vi "Photocell Read.vi"(0 "Arduino Resource":T1={"VISA resource"="", "Board Type"=enum."Arduino Uno", "Connection Type"=enum."USB / Serial", "Bytes Per Packet (15)"=15}, 5 "Photo Cell Pin (0)":u8, 9 "Vcc (5)":dbl=5.0, 11 "error in":errorcluster) -> (4 "Arduino Resource":T1={"VISA resource"="", "Board Type"=enum."Arduino Uno", "Connection Type"=enum."USB / Serial", "Bytes Per Packet (15)"=15}, 8 "Light Intensity (0 - 100)":dbl(knob) scale=0.0..100.0, 15 "error out":errorcluster)   [LabVIEW 2011, in "LabVIEW Interface for Arduino.lvlib"]
doc: "Measure light intensity using a Photocell. The user must specify the supply voltage (Vcc) in volts and the paired resistance in (R1) in Ohms. Light intensity is returned in arbitrary units and ranges from 0 in complete darkness to 100 in full direct light."
uses:
  LabVIEW Interface for Arduino.lvlib
  Private/Type Defs/Arduino Resource.ctl
  Private/Type Defs/Board Type.ctl
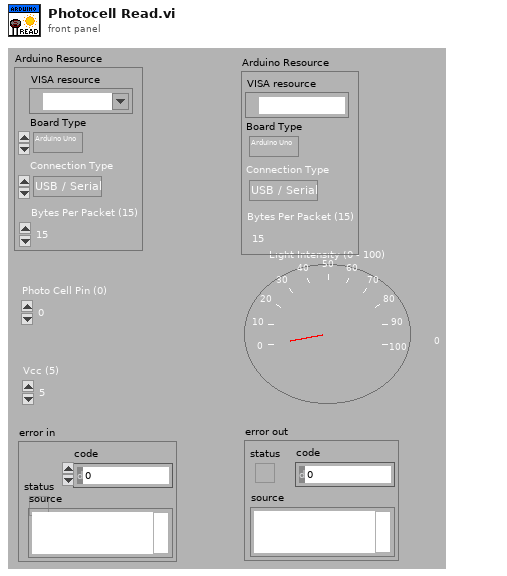
[diagram p1: front panel]
types:
  T1 = typedef "LabVIEW Interface for Arduino.lvlib/Arduino Resource.ctl" = cluster{"VISA resource":refnum<visa-resource-name>, "Board Type":T2, "Connection Type":enum8{"USB / Serial"}, "Bytes Per Packet (15)":u8}
  T2 = typedef "LabVIEW Interface for Arduino.lvlib/Board Type.ctl" = enum16{"Arduino Uno", "Dimuelanove w/Atmega 328", "Mega 2560", "Chipkit Uno32", "Chipkit Max32"}
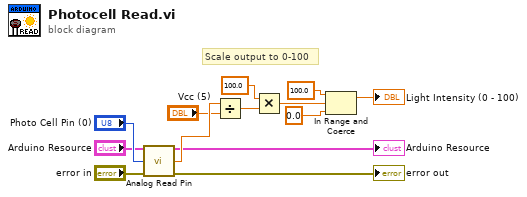
[diagram p0: block diagram]
diagram:
  # "Scale output to 0-100"
  n1 = call "Analog Read Pin.vi"("Arduino Resource"="Arduino Resource", "Analog Pin"="Photo Cell Pin (0)", "error in"="error in") -> ("Arduino Resource"=→"Arduino Resource":T1, "Voltage"=w11:dbl, "error out"=→"error out":errorcluster)  [unwired: 10 in]
  n2 = Divide(x=w11, y="Vcc (5)") -> (x/y=w10:dbl)
  n3 = Multiply(x=100.0, y=w10) -> (x*y=w4:dbl)
  n4 = In Range and Coerce(upper limit=100.0, x=w4, lower limit=0.0) -> (coerced(x)=→"Light Intensity (0 - 100)":dbl)  [unwired: 1 out]
